vi "FROG_average_default.vi"() -> ()   [LabVIEW 2016]
uses:
  <instrlib>/Ocean Optics 2000 4000/Ocean Optics 2000 4000.lvlib
panel:
  in  "Integration Time (6000us)":u32=6000
  in  "Average #":i32=5
  out "Spectral Waveform":cluster{dbl[], dbl[]}(graph)
  out "0.5*Max intens":dbl=4438.0
  in  "Final Position, mm":ext=21.35
  out "Pulse":dbl[][](graph)
  in  "Start FROG":bool
  in  "Enable Strobe (Disabled)":bool
  in  "VISA resource name":refnum<visa-resource-name>="USB0::0x2457::0x1012::NI-VISA-10001::RAW"
  in  "Initial Position, mm":ext=21.299999999999999999
  in  "Step Size, mm":ext=0.0001
  in  "MG17Motor":refnum<k7>(container)
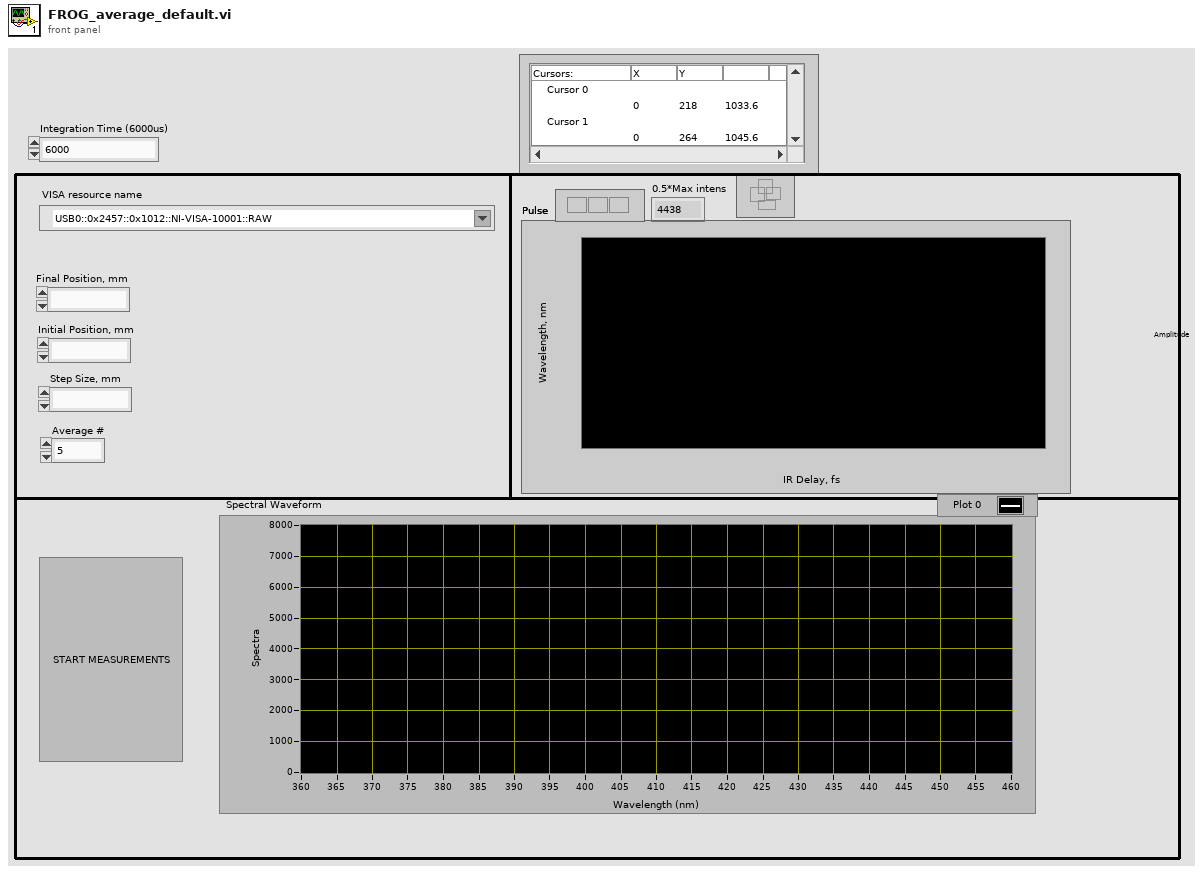
[diagram p1: front panel]
types:
  T1 = cluster{"Wavelength (nm)":dbl[], "Spectrum by Pixel Number":dbl[]}
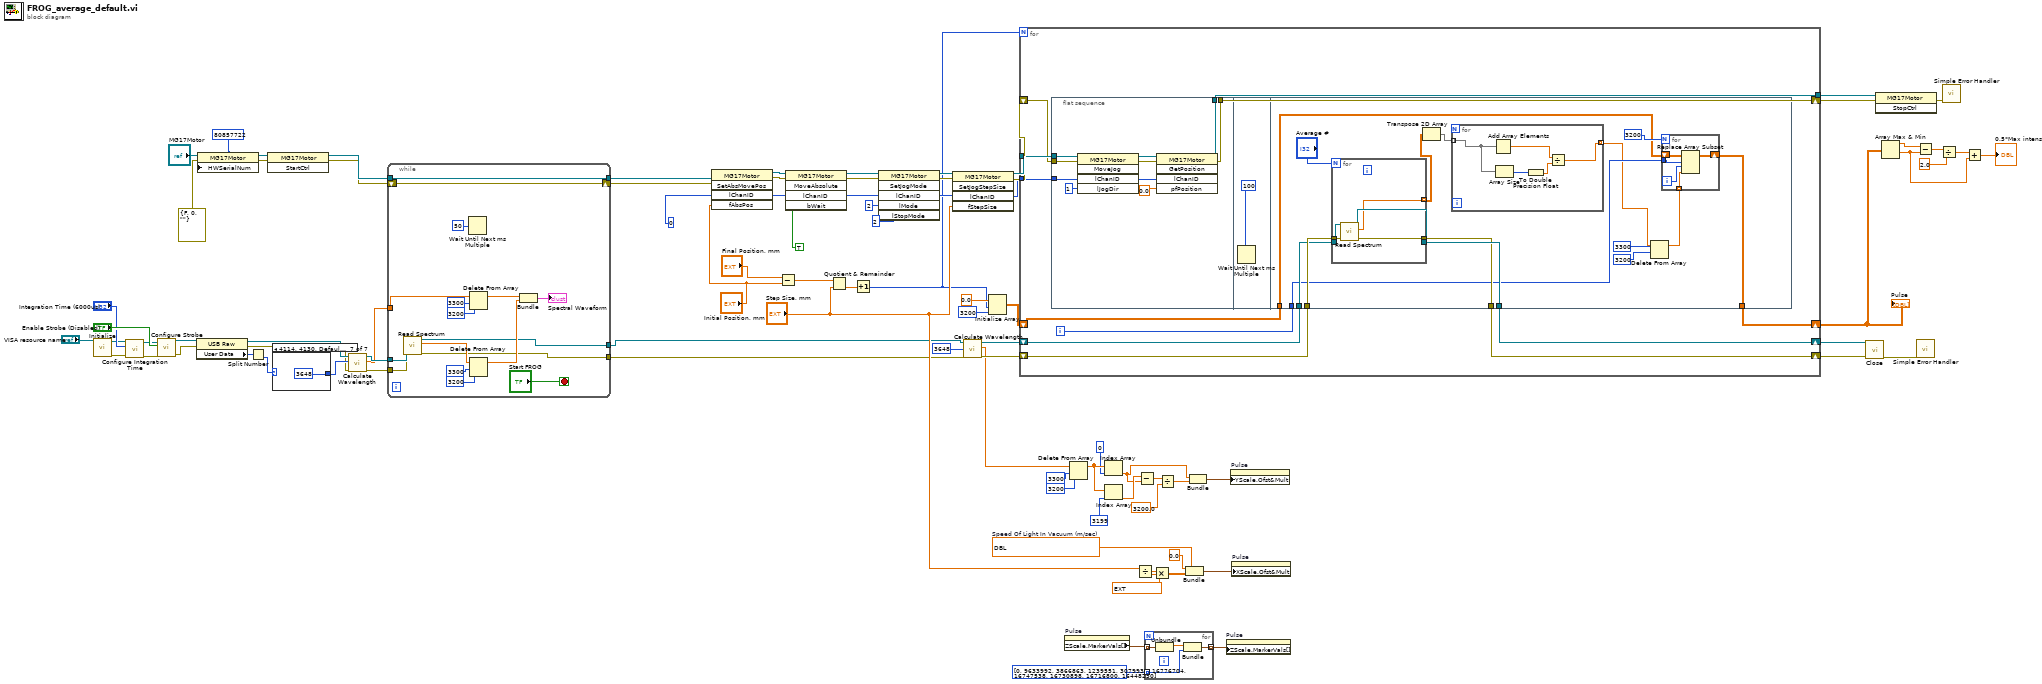
[diagram p0: block diagram]
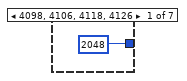
[diagram p2: hidden frame]
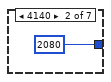
[diagram p3: hidden frame]
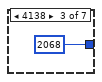
[diagram p4: hidden frame]
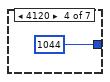
[diagram p5: hidden frame]
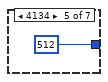
[diagram p6: hidden frame]
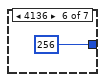
[diagram p7: hidden frame]
diagram:
  w79 = ext[unit] 299792458.0  # Speed Of Light In Vacuum (m/sec)
  n1 = call <instrlib>:"Initialize.vi"("VISA resource name"="VISA resource name") -> ("error out"=w3:errorcluster, "VISA resource name out"=w4:refnum<visa-resource-name>)  [unwired: 2 in, 7 out]
  n2 = call <instrlib>:"Configure Integration Time.vi"("error in (no error)"=w3, "Integration Time (6000)"="Integration Time (6000us)", "VISA resource name"=w4) -> ("error out"=w2:errorcluster, "VISA resource name out"=w1:refnum<visa-resource-name>)  [unwired: 7 out]
  n3 = call <instrlib>:"Configure Strobe.vi"("error in (no error)"=w2, "Enable Strobe (Disabled)"="Enable Strobe (Disabled)", "VISA resource name"=w1) -> ("error out"=w25:errorcluster, "VISA resource name out"=w24:refnum<visa-resource-name>)  [unwired: 7 out]
  n4 = property class="USB Raw"(reference=w24, error in=w25) -> (reference out=w22:refnum<visa-resource-name>, error out=w21:errorcluster, "User Data"=w50:u32)
  n5 = property class="MG17Motor"(reference="MG17Motor", error in=errorcluster {"status"=FALSE, "code"=0, "source"=""} ("error in (no error)"), "HWSerialNum"=80857722) -> (reference out=w67:refnum<k7>, error out=w66:errorcluster)
  n6 = Split Number(x=w50) -> (lo(x)=w49:u16)  [unwired: 1 out]
  n7 = invoke class="MG17Motor" method="StartCtrl"(reference=w67, error in=w66) -> (reference out=w45:refnum<k7>, error out=w44:errorcluster)  [unwired: 1 in, 1 out]
  n8 = case shown="4114, 4130, Default" w49 {
    tunnel: [2048 ("Number of Pixels (3840)") 2080 ("Number of Pixels (3840)") 2068 ("Number of Pixels (3840)") 1044 ("Number of Pixels (3840)") 512 ("Number of Pixels (3840)") 256 ("Number of Pixels (3840)") 3648 ("Number of Pixels (3840)")] -> w23
    frame 4098, 4106, 4118, 4126 {
    }
    frame 4140 {
    }
    frame 4138 {
    }
    frame 4120 {
    }
    frame 4134 {
    }
    frame 4136 {
    }
    frame 4114, 4130, Default {
    }
  }
  n9 = call <instrlib>:"Calculate Wavelength.vi"("error in (no error)"=w21, "Number of Pixels (3648)"=w23, "VISA resource name"=w22) -> ("error out"=w19:errorcluster, "Wavelength (nm)"=w6:dbl[], "VISA resource name out"=w20:refnum<visa-resource-name>)  [unwired: 6 out]
  n10 = while {
    tunnel: w45 -> [w113]
    tunnel: [w113] -> w9
    tunnel: w20 -> [w105]
    tunnel: w19 -> [w104]
    tunnel: w6 -> [w103]
    tunnel: [w99] -> w17
    tunnel: [w98] -> w16
    shift-right: [w112] -> w8
    shift-left: w44 -> [w112]
    stop <- "Start FROG" stop-if-true
    n11 = call <instrlib>:"Read Spectrum.vi"("error in (no error)"=w104, "VISA resource name"=w105) -> ("error out"=w98:errorcluster, "Spectrum by Pixel Number"=w101:dbl[], "VISA resource name out"=w99:refnum<visa-resource-name>)  [unwired: 6 in, 1 out]
    n12 = Wait Until Next ms Multiple(millisecond multiple=u32 50) -> ()  [unwired: 1 out]
    n13 = Delete From Array(array=w101, length=3300, index=3200) -> (array with subset deleted=w102:dbl[])  [unwired: 1 out]
    n14 = Delete From Array(array=w103, length=3300, index=3200) -> (array with subset deleted=w106:dbl[])  [unwired: 1 out]
    n15 = Bundle("Wavelength (nm)"=w106, "Spectrum by Pixel Number"=w102) -> (→"Spectral Waveform":T1)  [unwired: 1 out]
  }
  n16 = invoke class="MG17Motor" method="SetAbsMovePos"(reference=w9, error in=w8, "lChanID"=0, "fAbsPos"="Initial Position, mm") -> (reference out=w59:refnum<k7>, error out=w58:errorcluster, "lChanID"=w56:i32)  [unwired: 1 in, 2 out]
  n17 = Subtract(x="Final Position, mm", y="Initial Position, mm") -> (x-y=w40:ext)
  n18 = invoke class="MG17Motor" method="MoveAbsolute"(reference=w59, error in=w58, "lChanID"=w56, "bWait"=TRUE) -> (reference out=w48:refnum<k7>, error out=w47:errorcluster, "lChanID"=w55:i32)  [unwired: 1 in, 2 out]
  n19 = Quotient & Remainder(x=w40, y="Step Size, mm") -> (floor(x/y)=w39:ext)  [unwired: 1 out]
  n20 = Increment(x=w39) -> (x+1=w36:i32)
  n21 = invoke class="MG17Motor" method="SetJogMode"(reference=w48, error in=w47, "lChanID"=w55, "lMode"=2, "lStopMode"=2) -> (reference out=w64:refnum<k7>, error out=w62:errorcluster, "lChanID"=w54:i32)  [unwired: 1 in, 3 out]
  n22 = invoke class="MG17Motor" method="SetJogStepSize"(reference=w64, error in=w62, "lChanID"=w54, "fStepSize"="Step Size, mm") -> (reference out=w63:refnum<k7>, error out=w61:errorcluster, "lChanID"=w53:i32)  [unwired: 1 in, 2 out]
  n23 = call <instrlib>:"Calculate Wavelength.vi"("error in (no error)"=w16, "Number of Pixels (3648)"=3648, "VISA resource name"=w17) -> ("error out"=w14:errorcluster, "Wavelength (nm)"=w13:dbl[], "VISA resource name out"=w15:refnum<visa-resource-name>)  [unwired: 6 out]
  n24 = Initialize Array(0.0 ("element"), w36, 3200 ("dimension size")) -> (w35:dbl[][])
  n25 = for {
    N: w36 -> [_]
    tunnel: w63 -> [w126]
    tunnel: [w121] -> w43
    tunnel: w53 -> [w124]
    shift-right: [w119] -> w12
    shift-left: w15 -> [w123]
    shift-right: [w118] -> w11
    shift-left: w14 -> [w122]
    shift-right: [w115] -> w34
    shift-left: w35 -> [w117]
    shift-right: [w120] -> w57
    shift-left: w61 -> [w125]
    i -> [w116]
    n26 = flat-sequence {
      tunnel: w126 -> [w131]
      tunnel: w125 -> [w130]
      tunnel: w124 -> [w129]
      tunnel: [w127] -> w121
      tunnel: [w128] -> w120
      tunnel: w123 -> [w145]
      tunnel: w122 -> [w146]
      tunnel: [w143] -> w118
      tunnel: [w144] -> w119
      tunnel: w116 -> [w142]
      tunnel: w117 -> [w148]
      tunnel: [w147] -> w115
      frame #0 {
        n27 = invoke class="MG17Motor" method="MoveJog"(reference=w131, error in=w130, "lChanID"=w129, "lJogDir"=1) -> (reference out=w135:refnum<k7>, error out=w136:errorcluster, "lChanID"=w132:i32)  [unwired: 1 in, 2 out]
        n28 = invoke class="MG17Motor" method="GetPosition"(reference=w135, error in=w136, "lChanID"=w132, "pfPosition"=sgl 0.0) -> (reference out=w127:refnum<k7>, error out=w128:errorcluster)  [unwired: 1 in, 3 out]
      }
      frame #1 {
        n29 = Wait Until Next ms Multiple(millisecond multiple=u32 100) -> ()  [unwired: 1 out]
      }
      frame #2 {
        n30 = for {
          N: "Average #" -> [_]
          tunnel: [w158] -> w139 mode=indexing
          tunnel: w146 -> [w162]
          tunnel: [w159] -> w143
          tunnel: w145 -> [w161]
          tunnel: [w160] -> w144
          n31 = call <instrlib>:"Read Spectrum.vi"("error in (no error)"=w162, "VISA resource name"=w161) -> ("error out"=w159:errorcluster, "Spectrum by Pixel Number"=w158:dbl[], "VISA resource name out"=w160:refnum<visa-resource-name>)  [unwired: 6 in, 1 out]
        }
        n32 = Transpose 2D Array(2D array=w139) -> (transposed array=w138:dbl[][])
        n33 = for {
          tunnel: [w154] -> w140 mode=indexing
          tunnel: w138 -> [w153] mode=indexing
          n34 = Add Array Elements(numeric array=w153) -> (sum=w155:dbl)
          n35 = Array Size(array=w153) -> (size(s)=w157:i32)
          n36 = To Double Precision Float(number=w157) -> (double precision float=w156:dbl)
          n37 = Divide(x=w155, y=w156) -> (x/y=w154:dbl)
        }
        n38 = Delete From Array(array=w140, length=3200, index=3300) -> (array with subset deleted=w149:dbl[])  [unwired: 1 out]
        n39 = for {
          N: 3200 -> [_]
          shift-right: [w166] -> w147
          shift-left: w148 -> [w167]
          tunnel: w142 -> [w163]
          tunnel: w149 -> [w165] mode=indexing
          i -> [w164]
          n40 = Replace Array Subset(array=w167, new element=w165, index (row)=w163, index (col)=w164) -> (w166:dbl[][])
        }
      }
    }
  }
  "Pulse" <- w34
  n41 = property on="Pulse" class="IntGraph (strict)"() -> ("ZScale.MarkerVals[]"=w72:cluster{dbl, u32}[])  [unwired: 2 in, 2 out]
  n42 = Delete From Array(array=w13, length=3300, index=3200) -> (array with subset deleted=w88:dbl[])  [unwired: 1 out]
  n43 = Index Array(array=w88, index=0) -> (element=w80:dbl)
  n44 = Index Array(array=w88, index=3199) -> (element=w85:dbl)
  n45 = Divide(x="Step Size, mm", y=w79) -> (x/y=w78:ext)
  n46 = Subtract(x=w85, y=w80) -> (x-y=w83:dbl)
  n47 = for {
    tunnel: w72 -> [w171] mode=indexing
    tunnel: u32[] [0, 9633992, 3866863, 1239551, 3079936, 16776704, 16747538, 16730898, 16716800, 16448250] ("Custom Marker Colors 2") -> [w169] mode=indexing
    tunnel: [w168] -> w71 mode=indexing
    n48 = Unbundle(w171) -> (w170:dbl)  [unwired: 1 out]
    n49 = Bundle(w170, "Color Box"=w169) -> (w168:cluster{dbl, "Color Box":u32})  [unwired: 1 in]
  }
  n50 = Multiply(x=w78, y=ext 2000000000000.0) -> (x*y=w74:ext)
  n51 = Divide(x=w83, y=3200.0) -> (x/y=w82:dbl)
  n52 = Bundle(0.0, w74) -> (w75:cluster{dbl, ext})  [unwired: 1 in]
  n53 = Bundle(w80, w82) -> (w81:cluster{dbl, dbl})  [unwired: 1 in]
  n54 = property on="Pulse" class="IntGraph (strict)"("ZScale.MarkerVals[]"=w71) -> ()  [unwired: 2 in, 2 out]
  n55 = property on="Pulse" class="IntGraph (strict)"("YScale.Ofst&Mult"=w81) -> ()  [unwired: 2 in, 2 out]
  n56 = property on="Pulse" class="IntGraph (strict)"("XScale.Ofst&Mult"=w75) -> ()  [unwired: 2 in, 2 out]
  n57 = call <instrlib>:"Close.vi"("error in (no error)"=w11, "VISA resource name"=w12) -> ("error out"=w10:errorcluster)  [unwired: 9 out]
  n58 = invoke class="MG17Motor" method="StopCtrl"(reference=w43, error in=w57) -> (error out=w46:errorcluster)  [unwired: 1 in, 2 out]
  n59 = Array Max & Min(array=w34) -> (max value=w33:dbl, min value=w29:dbl)  [unwired: 2 out]
  n60 = call <vilib>:"Simple Error Handler.vi"("error in (no error)"=w10) -> ()  [unwired: 1 in, 8 out]
  n61 = Subtract(x=w33, y=w29) -> (x-y=w32:dbl)
  n62 = Divide(x=w32, y=2.0) -> (x/y=w30:dbl)
  n63 = call <vilib>:"Simple Error Handler.vi"("error in (no error)"=w46) -> ()  [unwired: 1 in, 8 out]
  n64 = Add(x=w30, y=w29) -> (x+y=→"0.5*Max intens":dbl)
